vi "VisChroma.vi"() -> ()   [LabVIEW 2018]
uses:
  AcPwrModule/PublicAPI/MeasurmentDataCluster.ctl
  <vilib>/Utility/error.llb/Error Cluster From Error Code.vi
  <vilib>/ErrorRing/Error Ring.xnode
  <userlib>/NIST/NISTErrorLib/NISTErrorLib.lvlib
  AcPwrPlugins.lvlib
panel:
  in  "Tab Control":enum32{"Chart", "XY Graph"}(tab)
  out "Chroma":waveform(dbl)[](graph)=[{"t0"=timestamp(3657200531.6397257 s since 1904-01-01), "dt"=1.0, "Y"=[46.19]}, {"t0"=timestamp(3657200531.6397257 s since 1904-01-01), "dt"=1.0, "Y"=[2.0]}, {"t0"=timestamp(3657200531.6397257 s since 1904-01-01), "dt"=1.0, "Y"=[60.0]}]
  in  "PlotYAxis":u32[](array[numeric])=[0, 1, 0] max=1
  out "Incorrect DataType?":bool
  out "Chroma's Internal Errors/Warnings":string="No Error"
  out "Current (A)":dbl(knob) scale=0.0..15.0
  out "Voltage (V)":dbl(knob) scale=0.0..100.0
  out "XY Graph":cluster{dbl[], dbl[]}(graph)={[0.02, 0.02, 0.02, 0.02, 0.02, 0.02, 0.02, 0.02, 0.1, 0.1, 0.1, 0.1, 0.1, 0.11, 0.2, 0.2, 0.2, 0.2, 0.2, 0.2, 0.3, 0.3, 0.3, 0.3, 0.3, 0.3, 0.3, 0.37, 0.4, 0.4, 0.4, 0.4, 0.4, 0.4, 0.48, 0.5, 0.5, 0.5, 0.5, 0.5, 0.5, 0.59, 0.6, 0.6, 0.6, 0.6, 0.6, 0.6, 0.6, 0.69, 0.69, 0.69, 0.69, 0.69, 0.69, 0.71, 0.79, 0.79, 0.79, 0.79, 0.79, 0.79, 0.89, 0.89, 0.89, 0.89, 0.89, 0.89, 0.89, 1.0, 1.0, 1.0, 1.0, 1.0, 1.0, 1.0, 1.1, 1.1, 1.1, 1.09, 1.09, 1.09, 1.1, 1.19, 1.19, 1.2, 1.2, 1.2, 1.2, 1.2, 1.29, 1.29, 1.29, 1.29, 1.29, 1.29, 1.29, 1.39, 1.39, 1.39, 1.39, 1.39, 1.39, 1.39, 1.4, 1.49, 1.49, 1.49, 1.49, 1.49, 1.49, 1.57, 1.59, 1.59, 1.59, 1.59, 1.59, 1.59, 1.69, 1.69, 1.69, 1.69, 1.69, 1.69, 1.69, 1.79, 1.79, 1.79, 1.79, 1.79, 1.79, 1.79, 1.89, 1.89, 1.89, 1.89, 1.89, 1.89, 1.89, 1.99, 1.99, 1.99, 1.99, 1.99, 1.99, 2.0, 2.09, 2.09, 2.09, 2.09, 2.09, 2.09, 2.13, 2.19, 2.19, 2.19, 2.19, 2.19, 2.19, 2.29, 2.29, 2.29, 2.29, 2.29, 2.29, 2.29, 2.29, 2.39, 2.39, 2.39, 2.39, 2.39, 2.39, 2.39, 2.49, 2.49, 2.49, 2.49, 2.49, 2.49, 2.51, 2.59, 2.59, 2.59, 2.59, 2.59, 2.59, 2.69, 2.69, 2.69, 2.69, 2.69, 2.69, 2.69, 2.79, 2.79, 2.79, 2.79, 2.79, 2.79, 2.79, 2.81, 2.89, 2.89, 2.89, 2.89, 2.89, 2.89, 2.89, 2.99, 2.99, 2.99, 2.99, 2.99, 2.99, 3.0, 3.09, 3.09, 3.09, 3.09, 3.09, 3.09, 3.1, 3.19, 3.19, 3.19, 3.19, 3.19, 3.19, 3.29, 3.29, 3.29, 3.29, 3.29, 3.29, 3.29, 3.39, 3.39, 3.39, 3.39, 3.39, 3.39, 3.39, 3.39, 3.49, 3.49, 3.49, 3.49, 3.49, 3.49, 3.49, 3.5, 3.59, 3.59, 3.59, 3.59, 3.59, 3.59, 3.6, 3.69, 3.69, 3.69, 3.69, 3.69, 3.69, 3.79, 3.79, 3.79, 3.79, 3.79, 3.79, 3.79, 3.89, 3.89, 3.89, 3.89, 3.89, 3.89, 3.89, 3.99, 3.99, 3.99, 3.99, 3.99, 3.99, 3.99], [42.02, 41.83, 42.15, 41.98, 41.52, 41.47, 41.64, 41.55, 41.51, 41.49, 41.46, 41.51, 41.41, 41.39, 41.42, 41.42, 41.41, 41.4, 41.29, 41.3, 41.32, 41.33, 41.32, 41.31, 41.32, 41.21, 41.21, 41.2, 41.2, 41.21, 41.22, 41.21, 41.1, 41.1, 41.09, 41.1, 41.09, 41.11, 41.1, 40.98, 40.99, 40.98, 40.98, 40.99, 40.99, 40.98, 40.98, 40.86, 40.86, 40.88, 40.87, 40.88, 40.87, 40.87, 40.74, 40.75, 40.75, 40.75, 40.73, 40.76, 40.63, 40.63, 40.62, 40.64, 40.64, 40.61, 40.64, 40.6, 40.5, 40.46, 40.5, 40.51, 40.5, 40.51, 40.37, 40.37, 40.37, 40.37, 40.37, 40.38, 40.37, 40.36, 40.22, 40.23, 40.23, 40.24, 40.23, 40.24, 40.1, 40.09, 40.07, 40.11, 40.09, 40.09, 40.11, 39.96, 39.96, 39.95, 39.96, 39.96, 39.96, 39.94, 39.81, 39.79, 39.79, 39.81, 39.8, 39.79, 39.79, 39.81, 39.65, 39.65, 39.65, 39.65, 39.64, 39.64, 39.65, 39.48, 39.48, 39.48, 39.48, 39.47, 39.48, 39.31, 39.31, 39.3, 39.31, 39.32, 39.31, 39.31, 39.14, 39.13, 39.13, 39.14, 39.13, 39.14, 39.13, 38.95, 38.95, 38.95, 38.94, 38.95, 38.95, 38.95, 38.75, 38.75, 38.76, 38.76, 38.75, 38.75, 38.75, 38.56, 38.56, 38.56, 38.56, 38.56, 38.55, 38.34, 38.34, 38.34, 38.33, 38.33, 38.34, 38.34, 38.11, 38.11, 38.1, 38.11, 38.12, 38.1, 38.11, 38.11, 37.87, 37.86, 37.86, 37.88, 37.86, 37.88, 37.86, 37.6, 37.61, 37.61, 37.61, 37.61, 37.61, 37.62, 37.33, 37.34, 37.33, 37.34, 37.34, 37.34, 37.04, 37.04, 37.05, 37.04, 37.06, 37.05, 37.04, 36.72, 36.72, 36.71, 36.72, 36.73, 36.72, 36.71, 36.72, 36.38, 36.37, 36.39, 36.37, 36.37, 36.38, 36.37, 36.0, 36.0, 35.99, 36.0, 35.99, 36.0, 35.99, 35.59, 35.59, 35.58, 35.58, 35.58, 35.58, 35.12, 35.12, 35.12, 35.13, 35.13, 35.13, 35.12, 34.6, 34.59, 34.59, 34.59, 34.59, 34.59, 34.59, 34.6, 33.97, 33.97, 33.98, 33.97, 33.98, 33.98, 33.98, 33.26, 33.27, 33.26, 33.26, 33.26, 33.26, 33.26, 33.26, 32.38, 32.39, 32.39, 32.37, 32.37, 32.39, 32.38, 31.25, 31.24, 31.25, 31.25, 31.25, 31.25, 29.64, 29.66, 29.66, 29.67, 29.65, 29.66, 29.66, 27.14, 27.15, 27.15, 27.15, 27.14, 27.14, 27.15, 17.86, 17.84]}
  in  "PluginName":string="AcPwr.Chroma0"
  out "ErrorArray":errorcluster[](array[cluster])
  in  "QueuName":string="CHROMADCVQ"
  in  "btnStop":bool
  in  "btnReset":bool
  in  "btnClear":bool
  # "0=Left Axis and 1=Right Axis"
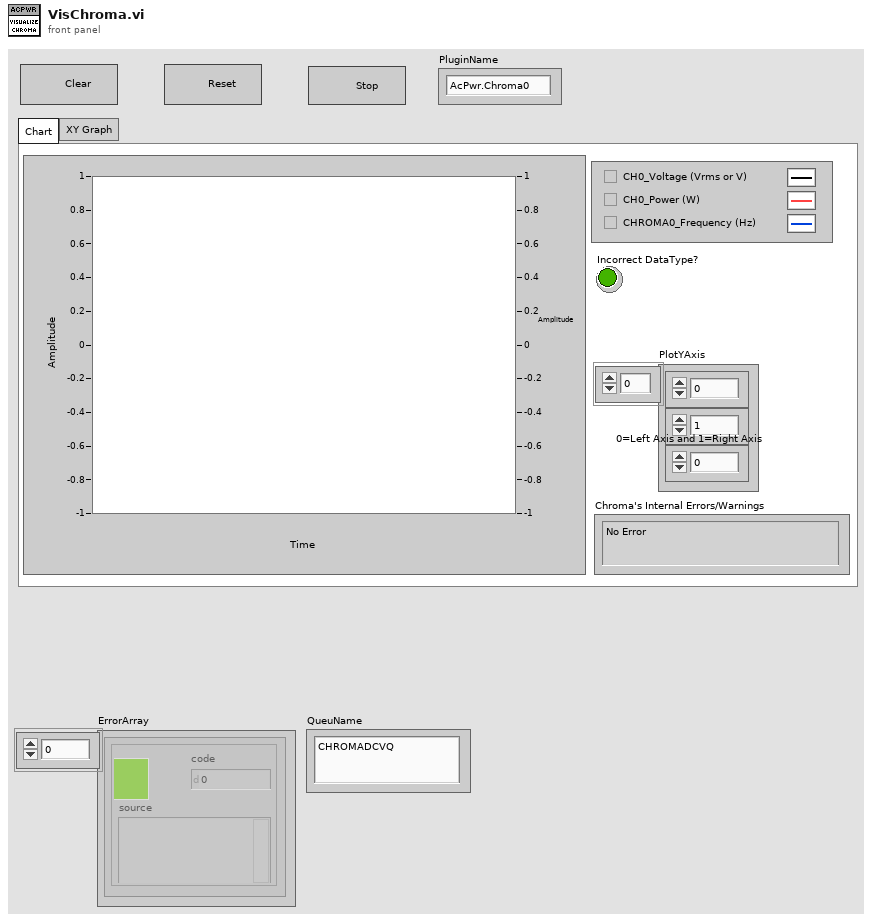
[diagram p1: front panel]
types:
  T1 = typedef "clBroadcastEvents.ctl" = cluster{"DidInit":refnum<user-event>, "StatusUpdate":refnum<user-event>, "ErrorReport":refnum<user-event>, "DidStop":refnum<user-event>, "PathToINI":refnum<user-event>, "Measurements":refnum<user-event>, "LoadConfigFile":refnum<user-event>, "GetSettings":refnum<user-event>, "SetSettings":refnum<user-event>, "GetType&ID":refnum<user-event>, "GotSettings":refnum<user-event>}
  T2 = typedef "MeasurmentDataCluster.ctl" = cluster{"MeasName":string, "XML Data":string, "WaveformData":waveform(dbl)[]}
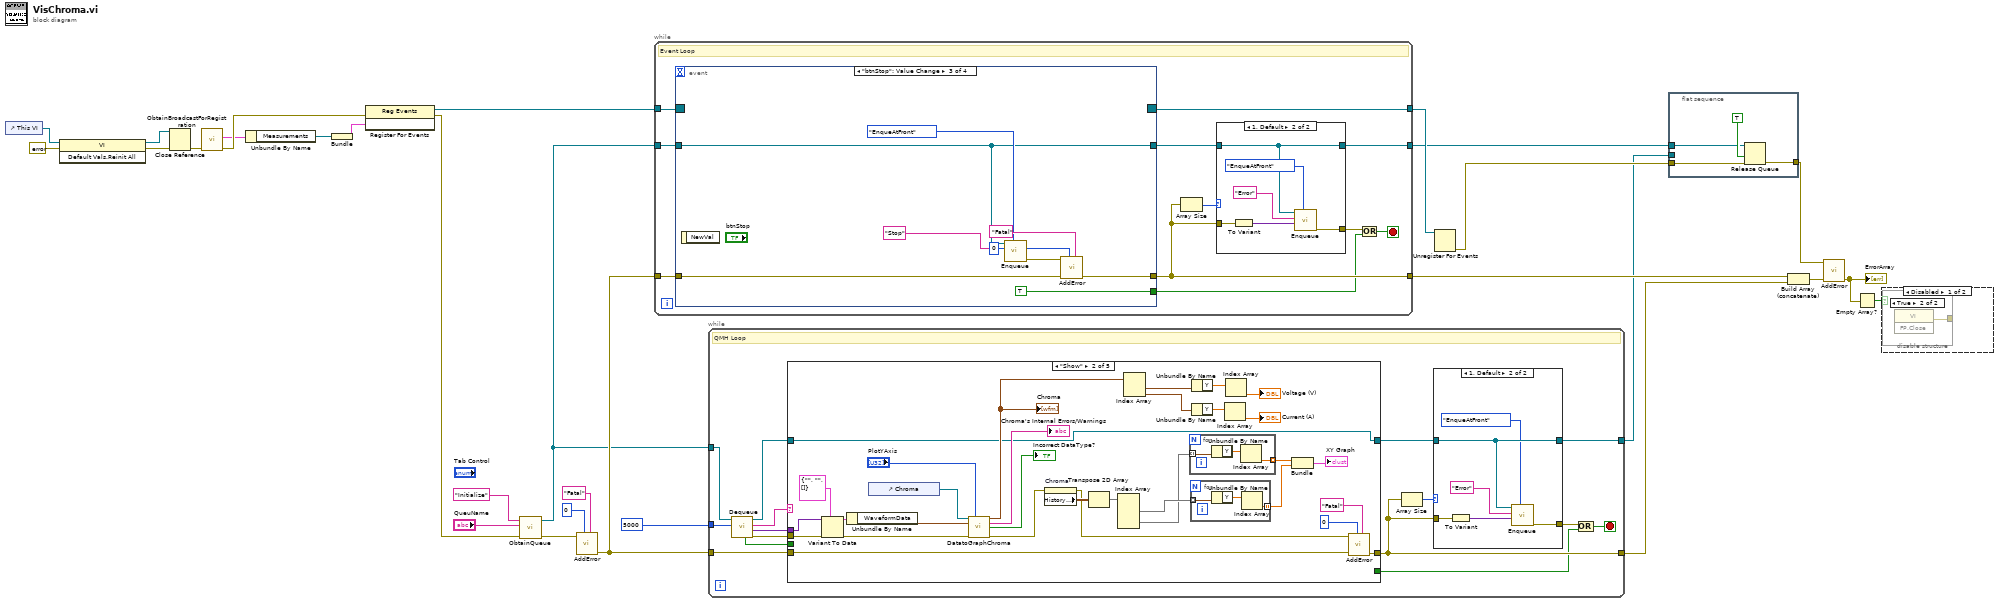
[diagram p0: block diagram]
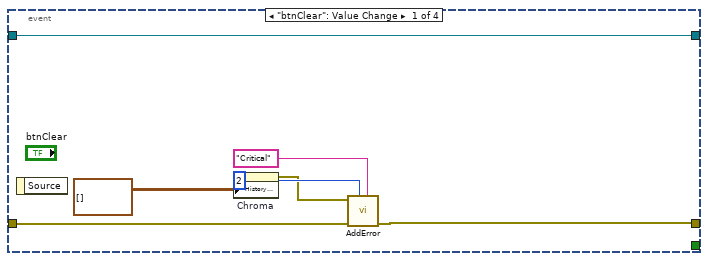
[diagram p5: hidden frame]
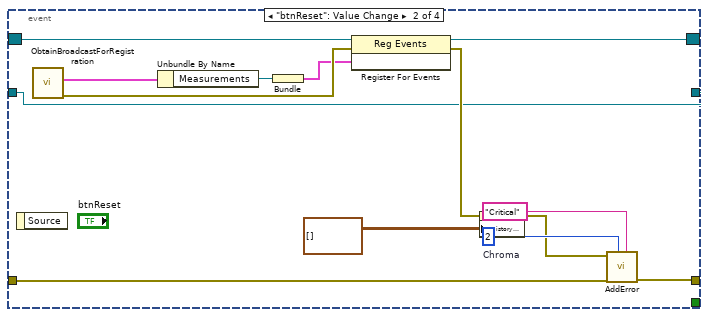
[diagram p6: hidden frame]
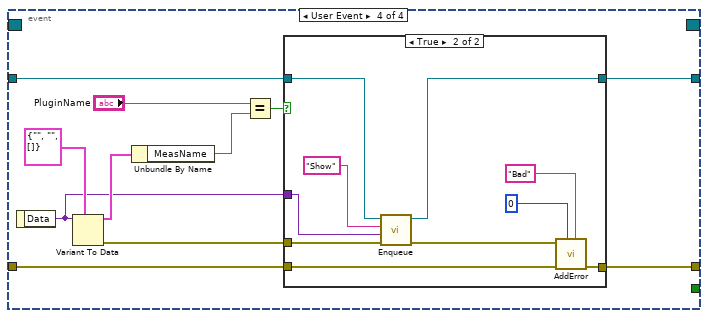
[diagram p7: hidden frame]
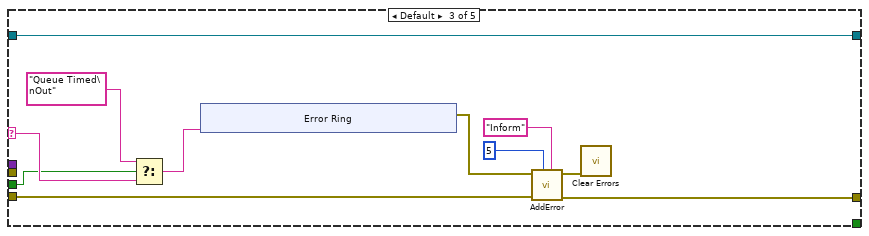
[diagram p11: hidden frame]
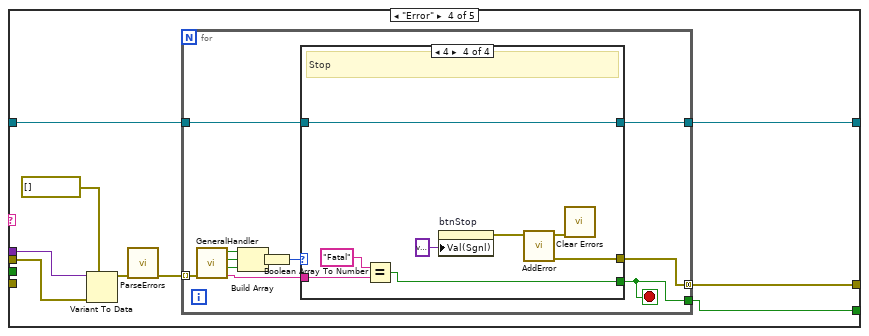
[diagram p12: hidden frame]
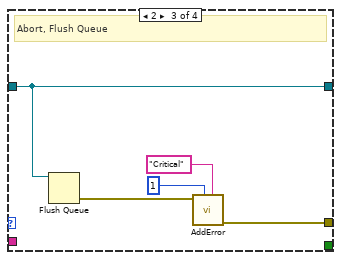
[diagram p15: hidden frame]
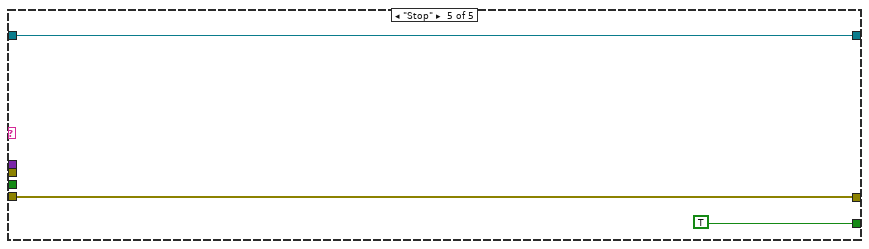
[diagram p16: hidden frame]
diagram:
  n1 = control-ref of="This VI"() -> (w19:refnum<vi>)
  n2 = invoke class="VI" method="Default Vals.Reinit All"(reference=w19, error in=errorcluster {"status"=FALSE, "code"=0, "source"=""} ("error in (no error)")) -> (reference out=w16:refnum<vi>, error out=w17:errorcluster)  [unwired: 1 in, 1 out]
  n3 = Close Reference(reference=w16, error in (no error)=w17) -> (error out=w15:errorcluster)
  n4 = call "ObtainBroadcastForRegistration.vi"("error in (no error)"=w15) -> ("error out"=w14:errorcluster, "clBroadcastEvents"=w13:T1)  [unwired: 9 in]
  n5 = Unbundle By Name(w13) -> ("Measurements"=w21:refnum<user-event>)
  n6 = Bundle("Measurements"=w21) -> (w20:cluster{"Measurements":refnum<user-event>})  [unwired: 1 in]
  n7 = register-events(error in=w14, w20) -> (reference out=w29:refnum<event-registration>, error out=w5:errorcluster)  [unwired: 1 in]
  n8 = call "ObtainQueue.vi"("error in (no error)"=w5, "ModuleName"="QueuName", "Initial Message"="Initialize" ("Message")) -> ("error out"=w8:errorcluster, "MessageQueue"=w4:refnum<queue>)  [unwired: 7 in]
  n9 = call <userlib>:"AddError.vi"("Severity"="Fatal", "Priority"=u8 0, "error in (no error)"=w8) -> ("ErrorArray"=w10:errorcluster[])  [unwired: 7 in, 1 out]
  n10 = while {
    tunnel: w29 -> [w40]
    tunnel: [w35] -> w27
    tunnel: [w39] -> w28
    tunnel: w10 -> [w38]
    tunnel: w4 -> [w37]
    tunnel: [w33] -> w3
    stop <- w30 stop-if-true
    # "Event Loop"
    n11 = event shown="[2] \"btnStop\": Value Change" {
      selector: w40 -> [_ w68 _ _]
      dyn-events: [_ w67 _ _] -> w39
      timeout: _ -> [_ _ _ _]
      tunnel: [_ _ TRUE _] -> w32
      tunnel: [w51 w62 w77 w88] -> w35
      tunnel: w38 -> [w52 w63 w71 w86]
      tunnel: w37 -> [w48 w55 w69 w83]
      tunnel: [w48 w55 w69 w82] -> w34
      event "btnClear": Value Change {
        n12 = event-data() -> ()  [unwired: 1 in, 1 out]
        n13 = property on="Chroma" class="WFChart (strict)"("History Data"=waveform(dbl)[][] []) -> (error out=w50:errorcluster)  [unwired: 2 in, 1 out]
        n14 = call <userlib>:"AddError.vi"("Severity"="Critical", "Priority"=u8 2, "ErrorArray"=w52, "error in (no error)"=w50) -> ("ErrorArray"=w51:errorcluster[])  [unwired: 6 in, 1 out]
      }
      event "btnReset": Value Change {
        n15 = event-data() -> ()  [unwired: 1 in, 1 out]
        n16 = call "ObtainBroadcastForRegistration.vi"() -> ("error out"=w64:errorcluster, "clBroadcastEvents"=w65:T1)  [unwired: 10 in]
        n17 = Unbundle By Name(w65) -> ("Measurements"=w66:refnum<user-event>)
        n18 = Bundle("Measurements"=w66) -> (w56:cluster{"Measurements":refnum<user-event>})  [unwired: 1 in]
        n19 = register-events(reference=w68, error in=w64, w56) -> (reference out=w67:refnum<event-registration>, error out=w58:errorcluster)
        n20 = property on="Chroma" class="WFChart (strict)"(error in=w58, "History Data"=waveform(dbl)[][] []) -> (error out=w57:errorcluster)  [unwired: 1 in, 1 out]
        n21 = call <userlib>:"AddError.vi"("Severity"="Critical", "Priority"=u8 2, "ErrorArray"=w63, "error in (no error)"=w57) -> ("ErrorArray"=w62:errorcluster[])  [unwired: 6 in, 1 out]
      }
      event "btnStop": Value Change {
        n22 = event-data() -> ()  [unwired: 1 in, 1 out]
        n23 = call "Enqueue.vi"("EnqueType (Enque)"=enum16{"LossyEnque", "EnqueAtFront", "Enque"}."EnqueAtFront", "Message"="Stop", "MessageQueue"=w69) -> ("error out"=w72:errorcluster)  [unwired: 7 in, 1 out]
        n24 = call <userlib>:"AddError.vi"("Severity"="Fatal" ("String"), "Priority"=u8 0, "ErrorArray"=w71, "error in (no error)"=w72) -> ("ErrorArray"=w77:errorcluster[])  [unwired: 6 in, 1 out]
      }
      event User Event {
        n25 = event-data() -> ("Data"=w78:variant)  [unwired: 1 in]
        n26 = Variant To Data(type=T2 {"MeasName"="", "XML Data"="", "WaveformData"=[]} ("MeasurmentDataCluster"), Variant=w78) -> (data=w80:T2, error out=w85:errorcluster)  [unwired: 1 in]
        n27 = Unbundle By Name(w80) -> ("MeasName"=w79:string)
        n28 = Equal?(x="PluginName", y=w79) -> (x = y?=w87:bool)
        n29 = case shown="True" w87 {
          tunnel: [w90 w97] -> w88
          tunnel: w86 -> [w90 w98]
          tunnel: w85 -> [_ w94]
          tunnel: w83 -> [w89 w93]
          tunnel: [w89 w92] -> w82
          tunnel: w78 -> [_ w91]
          frame False {
          }
          frame True {
            n30 = call "Enqueue.vi"("error in (no error)"=w94, "Message Data"=w91, "Message"="Show", "MessageQueue"=w93) -> ("error out"=w95:errorcluster, "MessageQueue"=w92:refnum<queue>)  [unwired: 6 in]
            n31 = call <userlib>:"AddError.vi"("Severity"="Bad" ("String"), "Priority"=u8 0, "ErrorArray"=w98, "error in (no error)"=w95) -> ("ErrorArray"=w97:errorcluster[])  [unwired: 6 in, 1 out]
          }
        }
      }
    }
    n32 = Array Size(array=w35) -> (size(s)=w36:i32)
    n33 = case shown="1, Default" w36 {
      tunnel: [_ w42] -> w31
      tunnel: w35 -> [_ w47]
      tunnel: w34 -> [w41 w44]
      tunnel: [w41 w44] -> w33
      frame 0 {
      }
      frame 1, Default {
        n34 = To Variant(anything=w47) -> (Variant=w46:variant)
        n35 = call "Enqueue.vi"("EnqueType (Enque)"=enum16{"LossyEnque", "EnqueAtFront", "Enque"}."EnqueAtFront", "Message Data"=w46, "Message"="Error", "MessageQueue"=w44) -> ("error out"=w42:errorcluster)  [unwired: 6 in, 1 out]
      }
    }
    n36 = Or(x=w31, y=w32) -> (x .or. y?=w30:bool)
  }
  n37 = while {
    tunnel: w10 -> [w113]
    tunnel: [w108] -> w9
    tunnel: w4 -> [w114]
    tunnel: [w106] -> w2
    tunnel: 5000 ("timeout in ms (-1)") -> [w104]
    stop <- w101 stop-if-true
    # "QMH Loop"
    n38 = call "Dequeue.vi"("timeout in ms (-1)"=w104, "MessageQueue"=w114) -> ("error out"=w111:errorcluster, "Message Data"=w115:variant, "Message"=w110:string, "MessageQueue"=w112:refnum<queue>, "timed out?"=w105:bool)  [unwired: 5 in]
    n39 = case shown="\"Show\"" w110 {
      selector: w110 -> [_ _ w165 _ _]
      tunnel: w115 -> [_ w133 _ w188 _]
      tunnel: w113 -> [w124 w153 w171 _ w216]
      tunnel: [w124 w155 w170 w184 w216] -> w108
      tunnel: [_ _ _ w183 TRUE] -> w102
      tunnel: w112 -> [w123 w127 w166 w182 w215]
      tunnel: w111 -> [_ w128 _ w181 _]
      tunnel: [w123 w127 w166 w180 w215] -> w109
      tunnel: w105 -> [_ _ w162 _ _]
      frame "Initialize" {
      }
      frame "Show" {
        n40 = Variant To Data(error in=w128, type=T2 {"MeasName"="", "XML Data"="", "WaveformData"=[]} ("MeasurmentDataCluster"), Variant=w133) -> (data=w131:T2, error out=w132:errorcluster)
        n41 = Unbundle By Name(w131) -> ("WaveformData"=w125:waveform(dbl)[])
        n42 = control-ref of="Chroma"() -> (w154:refnum<vi>)
        n43 = call "DatatoGraphChroma.vi"("WaveformChartReference"=w154, "PlotYScale"="PlotYAxis", "WaveformArray 2"=w125, "error in (no error)"=w132) -> ("WaveformArray"=w140:waveform(dbl)[], "OutputString"=→"Chroma's Internal Errors/Warnings":string, "Incorrect DataType?"=→"Incorrect DataType?":bool, "error out"=w148:errorcluster)  [unwired: 8 in]
        "Chroma" <- w140
        n44 = property on="Chroma" class="WFChart (strict)"(error in=w148) -> (error out=w129:errorcluster, "History Data"=w146:waveform(dbl)[][])  [unwired: 1 in, 1 out]
        n45 = Transpose 2D Array(2D array=w146) -> (transposed array=w147:waveform(dbl)[][])
        n46 = Index Array(array=w147) -> (element #1=w143:waveform(dbl)[], element #2=w142:waveform(dbl)[])  [unwired: 4 in]
        n47 = Index Array(array=w140) -> (element #1=w139:waveform(dbl), element #2=w138:waveform(dbl))  [unwired: 2 in]
        n48 = for {
          tunnel: w142 -> [w161] mode=indexing
          tunnel: [w159] -> w144 mode=indexing
          n49 = Unbundle By Name(w161) -> ("Y"=w160:dbl[])
          n50 = Index Array(array=w160) -> (element=w159:dbl)  [unwired: 1 in]
        }
        n51 = for {
          tunnel: w143 -> [w158] mode=indexing
          tunnel: [w156] -> w145 mode=indexing
          n52 = Unbundle By Name(w158) -> ("Y"=w157:dbl[])
          n53 = Index Array(array=w157) -> (element=w156:dbl)  [unwired: 1 in]
        }
        n54 = Unbundle By Name(w139) -> ("Y"=w137:dbl[])
        n55 = Unbundle By Name(w138) -> ("Y"=w136:dbl[])
        n56 = Index Array(array=w136) -> (element=→"Current (A)":dbl)  [unwired: 1 in]
        n57 = Index Array(array=w137) -> (element=→"Voltage (V)":dbl)  [unwired: 1 in]
        n58 = Bundle(w144, w145) -> (→"XY Graph":cluster{dbl[], dbl[]})  [unwired: 1 in]
        n59 = call <userlib>:"AddError.vi"("Severity"="Fatal" ("String"), "Priority"=u8 0, "ErrorArray"=w153, "error in (no error)"=w129) -> ("ErrorArray"=w155:errorcluster[])  [unwired: 6 in, 1 out]
      }
      frame Default {
        n60 = Select(t="Queue Timed\nOut", s=w162, f=w165) -> (s? t:f=w164:string)
        n61 = xnode "Error Ring"("parameter 0"=w164) -> ("error out"=w172:errorcluster)
        n62 = call <userlib>:"AddError.vi"("Severity"="Inform" ("String"), "Priority"=u8 5, "ErrorArray"=w171, "error in (no error)"=w172) -> ("ErrorArray"=w170:errorcluster[], "error out"=w169:errorcluster)  [unwired: 6 in]
        n63 = call <vilib>:"Clear Errors.vi"("error in (no error)"=w169) -> ()  [unwired: 5 in, 2 out]
      }
      frame "Error" {
        n64 = Variant To Data(error in=w181, type=errorcluster[] [], Variant=w188) -> (data=w186:errorcluster[])  [unwired: 1 out]
        n65 = call <userlib>:"ParseErrors.vi"("ErrorArray"=w186) -> ("ErrorArray"=w185:errorcluster[])  [unwired: 8 in, 2 out]
        n66 = for {
          tunnel: w185 -> [w199] mode=indexing
          tunnel: [w193] -> w184 mode=concatenating
          tunnel: [w191] -> w183
          tunnel: w182 -> [w190]
          tunnel: [w189] -> w180
          stop <- w191 stop-if-true
          n67 = call <userlib>:"GeneralHandler.vi"("error in (no error)"=w199) -> ("Severity"=w192:string, "Stop"=w196:bool, "Abort"=w197:bool, "Continue"=w198:bool)  [unwired: 7 in]
          n68 = Build Array(w198, w197, w196) -> (w195:bool[])
          n69 = Boolean Array To Number(Boolean array=w195) -> (number=w194:u32)
          n70 = case shown="4" w194 {
            tunnel: [_ _ w206 w214] -> w193
            tunnel: w192 -> [_ _ _ w212]
            tunnel: [_ _ _ w210] -> w191
            tunnel: w190 -> [w200 w201 w202 w207]
            tunnel: [w200 w201 w202 w207] -> w189
            frame 0, Default {
              # "No Dialog"
            }
            frame 1 {
              # "Continue"
            }
            frame 2 {
              # "Abort, Flush Queue"
              n71 = Flush Queue(queue=w202) -> (error out=w205:errorcluster)  [unwired: 1 in, 2 out]
              n72 = call <userlib>:"AddError.vi"("Severity"="Critical" ("String"), "Priority"=u8 1, "error in (no error)"=w205) -> ("ErrorArray"=w206:errorcluster[])  [unwired: 7 in, 1 out]
            }
            frame 4 {
              # "Stop"
              n73 = Equal?(x="Fatal", y=w212) -> (x = y?=w210:bool)
              n74 = property on="btnStop" class="Bool"("Val(Sgnl)"=variant ("Value (Signaling)")) -> (error out=w209:errorcluster)  [unwired: 2 in, 1 out]
              n75 = call <userlib>:"AddError.vi"("error in (no error)"=w209) -> ("ErrorArray"=w214:errorcluster[], "error out"=w213:errorcluster)  [unwired: 9 in]
              n76 = call <vilib>:"Clear Errors.vi"("error in (no error)"=w213) -> ()  [unwired: 5 in, 2 out]
            }
          }
        }
      }
      frame "Stop" {
      }
    }
    n77 = Array Size(array=w108) -> (size(s)=w107:i32)
    n78 = case shown="1, Default" w107 {
      tunnel: [_ w117] -> w103
      tunnel: w108 -> [_ w122]
      tunnel: w109 -> [w116 w119]
      tunnel: [w116 w119] -> w106
      frame 0 {
      }
      frame 1, Default {
        n79 = To Variant(anything=w122) -> (Variant=w121:variant)
        n80 = call "Enqueue.vi"("EnqueType (Enque)"=enum16{"LossyEnque", "EnqueAtFront", "Enque"}."EnqueAtFront", "Message Data"=w121, "Message"="Error", "MessageQueue"=w119) -> ("error out"=w117:errorcluster)  [unwired: 6 in, 1 out]
      }
    }
    n81 = Or(x=w103, y=w102) -> (x .or. y?=w101:bool)
  }
  n82 = Unregister For Events(event registration refnum=w28) -> (error out=w26:errorcluster)  [unwired: 1 in]
  n83 = flat-sequence {
    tunnel: w26 -> [w218]
    tunnel: [w221] -> w24
    tunnel: w3 -> [w219]
    tunnel: w2 -> [_]
    frame #0 {
      n84 = Release Queue(queue=w219, force destroy? (F)=TRUE, error in (no error)=w218) -> (error out=w221:errorcluster)  [unwired: 2 out]
    }
  }
  n85 = Build Array (concatenate)(w27, w9) -> (w25:errorcluster[])
  n86 = call <userlib>:"AddError.vi"("ErrorArray"=w25, "error in (no error)"=w24) -> ("ErrorArray"=w23:errorcluster[])  [unwired: 8 in, 1 out]
  "ErrorArray" <- w23
  n87 = Empty Array?(array=w23) -> (empty?=w22:bool)
  n88 = disable-structure shown="Disabled" {
    disable-tunnel: w22 -> [w222 _]
    frame Disabled {
      n89 = case shown="True" w222 {
        tunnel: [_ w223] -> _
        frame False {
        }
        frame True {
          n90 = invoke class="VI" method="FP.Close"() -> (error out=w223:errorcluster)  [unwired: 3 in, 2 out]
        }
      }
    }
    frame Enabled {
    }
  }
